vi "Read Terminals and Acyclic Frame Names.vi"(8 "error in":errorcluster, 11 "port in":T1 format="%.0x") -> (0 "error out":errorcluster, 2 "terminals":T2[](array[typedef]), 3 "port out":T1 format="%.0x", 4 "acyclic frame names":string[](array[string]))   [LabVIEW 2020, in "Ballard MIL-STD-1553 Scripting.lvlib"]
uses:
  Ballard MIL-STD-1553 Scripting.lvlib
  Shared/Address.ctl
  Shared/Terminal Name and Address.ctl
  <vilib>/NI VeriStand/Custom Device Tools/Custom Device Utility Library/Custom Device Utility Library.lvlib
  Constants.vi
  <vilib>/NI VeriStand/Custom Device API/Custom Device API.lvlib
  <vilib>/NI VeriStand/Custom Device Tools/Custom Device Utility Library/NI VeriStand - Search for All Items by GUID.vi
  <vilib>/NI VeriStand/Custom Device API/Get Item Property (String).vi
  <vilib>/NI VeriStand/Custom Device API/Custom Device Item Ref.ctl
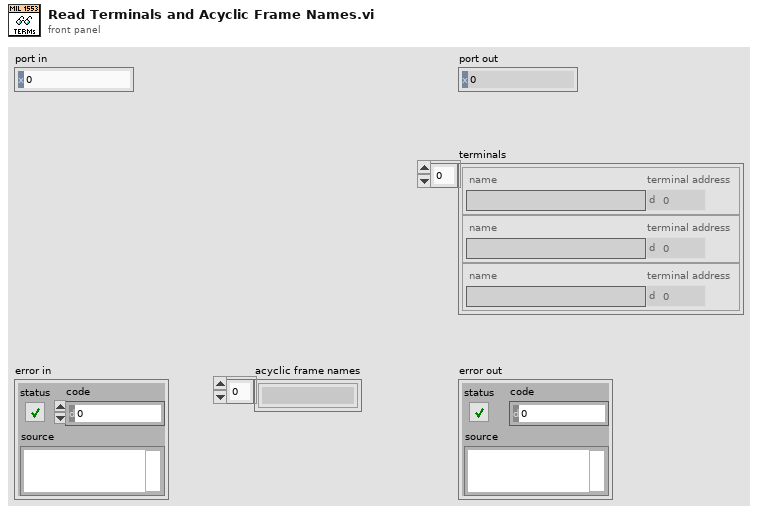
[diagram p1: front panel]
types:
  T1 = typedef "Custom Device API.lvlib/Custom Device Item Ref.ctl" = u64
  T2 = typedef "Terminal Name and Address.ctl" = cluster{"name":string, "terminal address":T3}
  T3 = typedef "Address.ctl" = u16
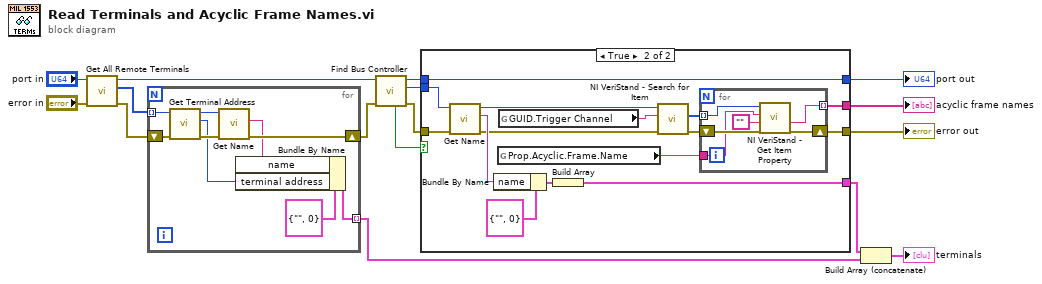
[diagram p0: block diagram]
diagram:
  n1 = call "Get All Remote Terminals.vi"("error in"="error in", "port in"="port in") -> ("error out"=w5:errorcluster, "remote terminals"=w7:T1[], "port out"=w10:T1)  [unwired: 7 in]
  n2 = for {
    shift-right: [w25] -> w11
    shift-left: w5 -> [w24]
    tunnel: w7 -> [w22] mode=indexing
    tunnel: [w18] -> w12 mode=indexing
    n3 = call "Get Terminal Address.vi"("error in"=w24, "remote terminal in"=w22) -> ("error out"=w21:errorcluster, "port number"=w19:u16, "remote terminal out"=w23:T1)  [unwired: 6 in, 1 out]
    n4 = call "Get Name.vi"("error in"=w21, "Ballard MIL-STD 1553 custom device in"=w23) -> ("error out"=w25:errorcluster, "name"=w20:string)  [unwired: 7 in, 1 out]
    n5 = Bundle By Name(cluster=T2 {"name"="", "terminal address"=0} ("terminal"), "name"=w20, "terminal address"=w19) -> (w18:T2)
  }
  n6 = call "Find Bus Controller.vi"("error in"=w11, "port in"=w10) -> ("error out"=w4:errorcluster, "bus controller"=w6:T1, "port out"=w2:T1, "found?"=w3:bool)  [unwired: 6 in]
  n7 = case shown="True" w3 {
    tunnel: w2 -> [w27 w41]
    tunnel: w4 -> [w26 w42]
    tunnel: [w27 w41] -> w1
    tunnel: [w26 w29] -> w15
    tunnel: w6 -> [_ w40]
    tunnel: [_ w36] -> w14
    tunnel: [_ w28] -> w16
    frame False {
    }
    frame True {
      n8 = call "Get Name.vi"("error in"=w42, "Ballard MIL-STD 1553 custom device in"=w40) -> ("error out"=w33:errorcluster, "name"=w38:string, "Ballard MIL-STD 1553 custom device out"=w35:T1)  [unwired: 7 in]
      n9 = Bundle By Name(cluster=T2 {"name"="", "terminal address"=0} ("terminal"), "name"=w38) -> (w37:T2)
      n10 = global read "Constants.vi" "Prop.Acyclic.Frame.Name"() -> (w30:string)
      n11 = global read "Constants.vi" "GUID.Trigger Channel"() -> (w34:string)
      n12 = Build Array(w37) -> (w36:T2[])
      n13 = call-poly <vilib>:"NI VeriStand - Search for Item.vi"("error in"=w33, "Item GUID"=w34, "Section Ref in"=w35) -> ("error out"=w31:errorcluster, "Item Refs"=w32:T1[])  [unwired: 5 in, 2 out]
      n14 = for {
        tunnel: w32 -> [w47] mode=indexing
        shift-right: [w48] -> w29
        shift-left: w31 -> [w46]
        tunnel: w30 -> [w45]
        tunnel: [w43] -> w28 mode=indexing
        n15 = call-poly <vilib>:"NI VeriStand - Get Item Property.vi"("error in (no error)"=w46, "Default Value"="", "Property Name"=w45, "Item Ref in"=w47) -> ("error out"=w48:errorcluster, "Value"=w43:string)  [unwired: 4 in, 2 out]
      }
    }
  }
  "acyclic frame names" <- w16
  "error out" <- w15
  "port out" <- w1
  n16 = Build Array (concatenate)(w14, w12) -> (→"terminals":T2[])
